vi "derivative.vi"(10 "Starting value":dbl, 11 "x":dbl) -> (3 "dx/dt":dbl)   [LabVIEW 2016]
doc: "Takes the derivative of the input with respect to real time"
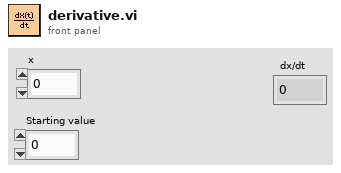
[diagram p1: front panel]
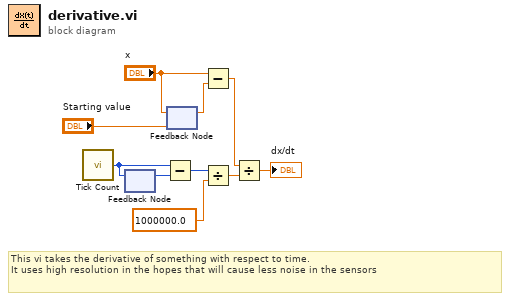
[diagram p0: block diagram]
diagram:
  # "This vi takes the derivative of something with respect to time.\nIt uses high resolution in the hopes that will cause less noise in the sensors"
  n1 = call "Tick Count"() -> ("Tick Count(uSec)"=w1:u32)
  n2 = feedback #1() -> (w6:u32)  [unwired: 1 in]
  n3 = feedback-in #1(w1) -> ()
  n4 = Subtract(x=w1, y=w6) -> (x-y=w4:u32)
  n5 = feedback #2("Starting value") -> (w10:dbl)
  n6 = feedback-in #2("x") -> ()
  n7 = Subtract(x="x", y=w10) -> (x-y=w8:dbl)
  n8 = Divide(x=w4, y=1000000.0) -> (x/y=w2:dbl)
  n9 = Divide(x=w8, y=w2) -> (x/y=→"dx/dt":dbl)
